vi "Resize.vi"(8 "error in (no error)":errorcluster, 11 "CollapsePanel in":refnum<class "CollapsePanel.lvclass">) -> (0 "error out":errorcluster, 3 "CollapsePanel out":refnum<class "CollapsePanel.lvclass">)   [LabVIEW 2021, in "CollapsePanel.lvclass"]
uses:
  CollapsePanel.lvclass
  CollapsePanel.lvclass/CollapsePanel.ctl
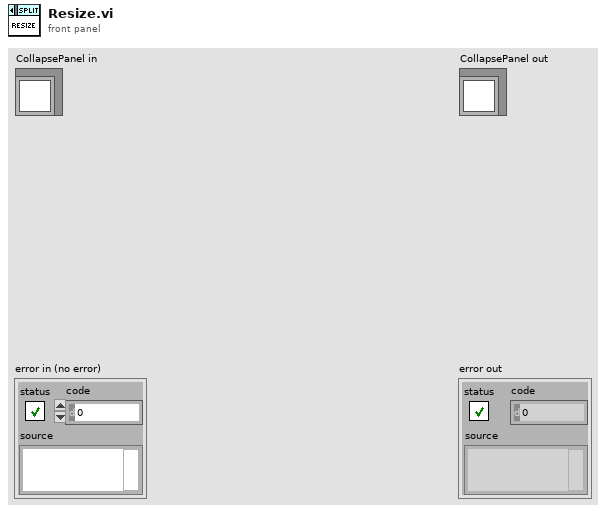
[diagram p1: front panel]
types:
  T1 = typedef "CollapsePanel.lvclass/collapse direction.ctl" = enum16{"Left", "Right", "Up", "Down"}
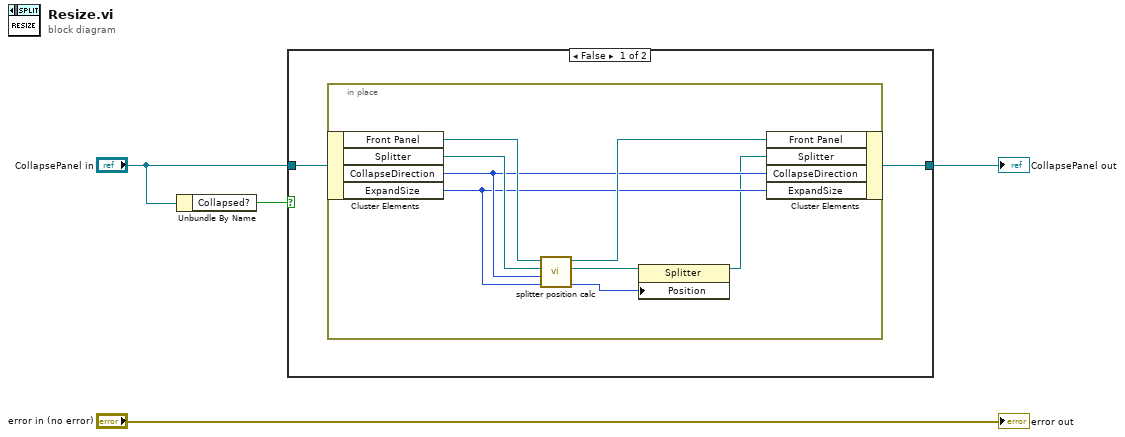
[diagram p0: block diagram]
diagram:
  n1 = Unbundle By Name("CollapsePanel in") -> ("Collapsed?"=w1:bool)
  n2 = case shown="False" w1 {
    tunnel: [w6 w15] -> w4
    tunnel: "CollapsePanel in" -> [w5 w15]
    frame False {
      n3 = in-place {
        n4 = in-place-cluster #1(w5) -> ("Front Panel"=w14:refnum<vi>, "Splitter"=w13:refnum<vi>, "CollapseDirection"=w11:T1, "ExpandSize"=w10:i32)
        n5 = call "splitter position calc.vi"("ExpandSize"=w10, "CollapseDirection"=w11, "Splitter"=w13, "Front Panel"=w14) -> ("Splitter Position"=w7:i32, "Splitter"=w9:refnum<vi>, "Front Panel"=w12:refnum<vi>)  [unwired: 5 in]
        n6 = property class="Splitter"(reference=w9, "Position"=w7) -> (reference out=w8:refnum<vi>)  [unwired: 1 in, 1 out]
        n7 = in-place-cluster #1("Front Panel"=w12, "Splitter"=w8, "CollapseDirection"=w11, "ExpandSize"=w10) -> (w6:refnum<class "CollapsePanel.lvclass">)
      }
    }
    frame True {
    }
  }
  "CollapsePanel out" <- w4
  "error out" <- "error in (no error)"
